vi "Energy Values.vi"(0 "power values":T2, 1 "reset? (F)":bool, 5 "energy accumulation":enum16{"Interval only", "Accumulated"}(ring), 7 "interval length [s]":dbl=0.2, 9 "system info in":refnum<class "EP System Info.lvclass">, 11 "error in (no error)":errorcluster) -> (4 "energy values":T1, 8 "accumulation length [s]":dbl, 10 "system info out":refnum<class "EP System Info.lvclass">, 15 "error out":errorcluster)   [LabVIEW 2014, in "NI_EP_Power Quality.lvlib"]
doc: "Calculates energy values for a specified interval length. This VI returns apparent, active, and reactive energy values.\n\nThis VI supports measuring single-line and multiple-line systems."
uses:
  <vilib>/addons/Electrical Power/PQ/NI_EP_Power Quality.lvlib
  <vilib>/addons/Electrical Power/PQ/Common/Classes/System Info/EP System Info.lvclass
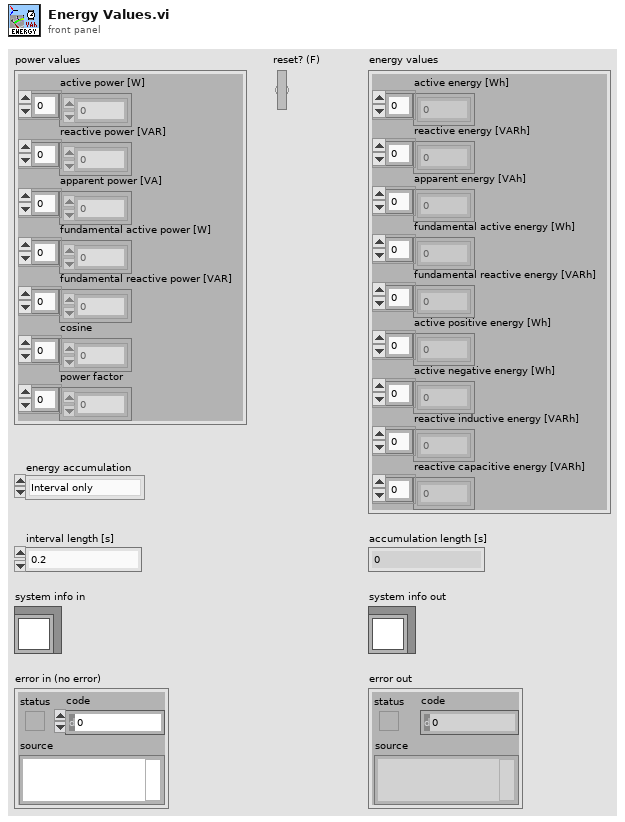
[diagram p1: front panel]
types:
  T1 = cluster{"active energy [Wh]":dbl[], "reactive energy [VARh]":dbl[], "apparent energy [VAh]":dbl[], "fundamental active energy [Wh]":dbl[], "fundamental reactive energy [VARh]":dbl[], "active positive energy [Wh]":dbl[], "active negative energy [Wh]":dbl[], "reactive inductive energy [VARh]":dbl[], "reactive capacitive energy [VARh]":dbl[]}
  T2 = cluster{"active power [W]":dbl[], "reactive power [VAR]":dbl[], "apparent power [VA]":dbl[], "fundamental active power [W]":dbl[], "fundamental reactive power [VAR]":dbl[], "cosine":dbl[], "power factor":dbl[]}
  T3 = cluster{"active power [W]":dbl[], "reactive power [VAR]":dbl[], "apparent power [VA]":dbl[], "fundamental active power [W]":dbl[], "fundamental reactive power [VAR]":dbl[], dbl[], dbl[], dbl[], dbl[]}
  T4 = cluster{"active energy AP (Wh)":dbl[], "reactive energy AQ (VArh)":dbl[], "apparent energy AS (VAh)":dbl[], "fundamental active energy AP1 (Wh)":dbl[], "fundamental reactive energy AQ1 (VArh)":dbl[], "active positive energy AP in (Wh)":dbl[], "active negative energy AP out (Wh)":dbl[], "reactive inductive energy AQL (VArh)":dbl[], "reactive capacitance energy AQC (VArh)":dbl[]}
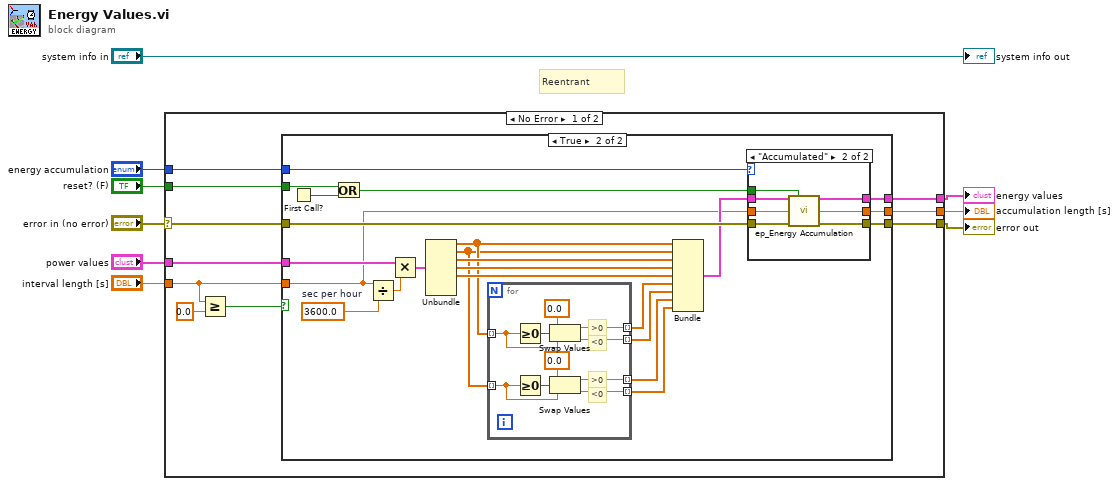
[diagram p0: block diagram]
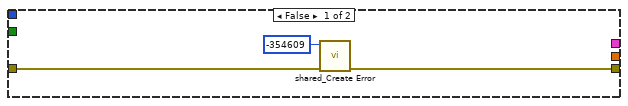
[diagram p2: hidden frame]
diagram:
  # "Reentrant"
  n1 = case shown="No Error" "error in (no error)" {
    selector: "error in (no error)" -> [w18 w66]
    tunnel: "power values" -> [w19 _]
    tunnel: "interval length [s]" -> [w12 _]
    tunnel: "energy accumulation" -> [w17 _]
    tunnel: [w16 _] -> w4
    tunnel: [w15 _] -> w3
    tunnel: [w14 w66] -> w2
    tunnel: "reset? (F)" -> [w13 _]
    frame No Error {
      n2 = Greater Or Equal?(x=w12, y=0.0) -> (x >= y?=w10:bool)
      n3 = case shown="True" w10 {
        tunnel: w19 -> [_ w44]
        tunnel: w18 -> [w22 w32]
        tunnel: w17 -> [_ w30]
        tunnel: [_ w29] -> w16
        tunnel: [_ w28] -> w15
        tunnel: w12 -> [_ w27]
        tunnel: [w21 w26] -> w14
        tunnel: w13 -> [_ w24]
        frame False {
          n4 = call <vilib>:"shared_Create Error.vi"("error in (no error)"=w22, "error code (0)"=-354609) -> ("error out"=w21:errorcluster)  [unwired: 9 in]
        }
        frame True {
          w45 = 3600.0  # sec per hour
          n5 = First Call?() -> (First Call?: T/F=w25:bool)
          n6 = Or(x=w24, y=w25) -> (x .or. y?=w23:bool)
          n7 = Divide(x=w27, y=w45) -> (x/y=w43:dbl)
          n8 = Multiply(x=w44, y=w43) -> (x*y=w42:T2)
          n9 = Unbundle(w42) -> ("active power [W]"=w38:dbl[], "reactive power [VAR]"=w33:dbl[], "apparent power [VA]"=w41:dbl[], "fundamental active power [W]"=w40:dbl[], "fundamental reactive power [VAR]"=w39:dbl[])  [unwired: 2 out]
          n10 = for {
            tunnel: w38 -> [w61] mode=indexing
            tunnel: w33 -> [w58] mode=indexing
            tunnel: [w63] -> w37 mode=indexing
            tunnel: [w62] -> w36 mode=indexing
            tunnel: [w57] -> w35 mode=indexing
            tunnel: [w56] -> w34 mode=indexing
            # "<0"
            # ">0"
            # "<0"
            # ">0"
            n11 = Greater Or Equal To 0?(x=w61) -> (x >= 0?=w65:bool)
            n12 = Greater Or Equal To 0?(x=w58) -> (x >= 0?=w59:bool)
            n13 = Swap Values(12:0.0 ("f"), 13:w65, 14:w61) -> (1:w63:dbl, 3:w62:dbl)
            n14 = Swap Values(12:0.0 ("f"), 13:w59, 14:w58) -> (1:w57:dbl, 3:w56:dbl)
          }
          n15 = Bundle("active power [W]"=w38, "reactive power [VAR]"=w33, "apparent power [VA]"=w41, "fundamental active power [W]"=w40, "fundamental reactive power [VAR]"=w39, w37, w36, w35, w34) -> (w31:T3)  [unwired: 1 in]
          n16 = case shown="\"Accumulated\"" w30 {
            tunnel: w32 -> [w46 w55]
            tunnel: w31 -> [w48 w54]
            tunnel: [w48 w53] -> w28
            tunnel: [w47 w49] -> w29
            tunnel: w27 -> [w47 w50]
            tunnel: [w46 w52] -> w26
            tunnel: w23 -> [_ w51]
            frame "Interval only", Default {
            }
            frame "Accumulated" {
              n17 = call <vilib>:"ep_Energy Accumulation.vi"("energy values"=w54, "restart (F)"=w51, "interval length (s)"=w50, "error in (no error)"=w55) -> ("accumulated energy"=w53:T4, "accumulation length (s)"=w49:dbl, "error out"=w52:errorcluster)  [unwired: 9 in]
            }
          }
        }
      }
    }
    frame Error {
    }
  }
  "error out" <- w2
  "energy values" <- w3
  "accumulation length [s]" <- w4
  "system info out" <- "system info in"
